vi "Trace Results.vi"(9 "Status of previous command":T1, 10 "Description":string, 11 "Subsystem":string) -> ()   [LabVIEW 2015]
doc: "This VI displays the execution trace of various commands and subsystems. Use command descriptions and controller print formatting to make it easier to understand the trace."
uses:
  <vilib>/Rock Robotics/WPI/Framework/Completion Status.ctl
panel:
  in  "Trace Enable":bool
  out "Subsystem Trace":T2(array[cluster])
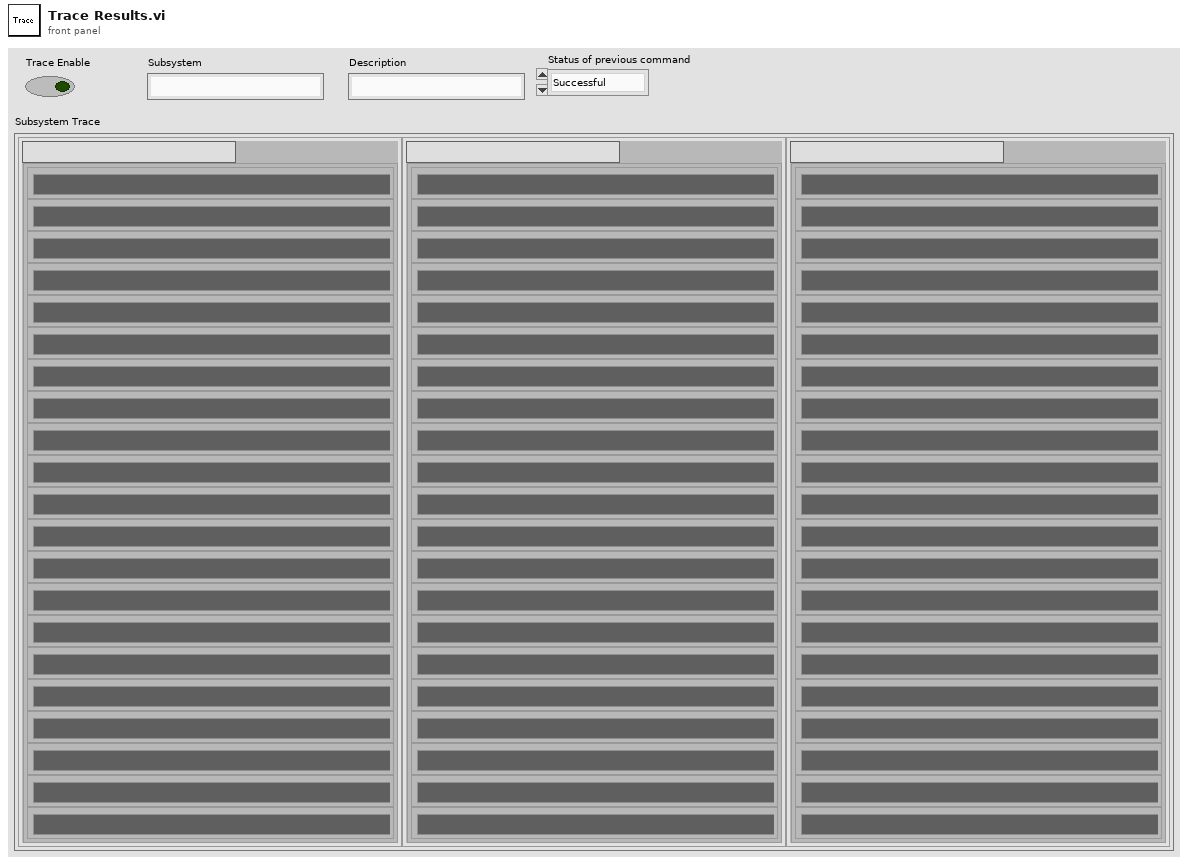
[diagram p1: front panel]
types:
  T1 = typedef "Completion Status.ctl" = enum16{"Successful", "Aborted", "Incomplete"}
  T2 = cluster{"Subsystem":string, "Tracings":cluster{"Command":string, "Color":u32}[]}[]
  T3 = cluster{"Subsystem":string, "Tracings":cluster{"Command":string, "Color":u32}[]}
  T4 = cluster{"Subsystem":string, cluster{"Description":string, "Active":u32}[]}
  T5 = cluster{"Subsystem":string, "Tracings":cluster{"Description":string, "Active":u32}[]}[]
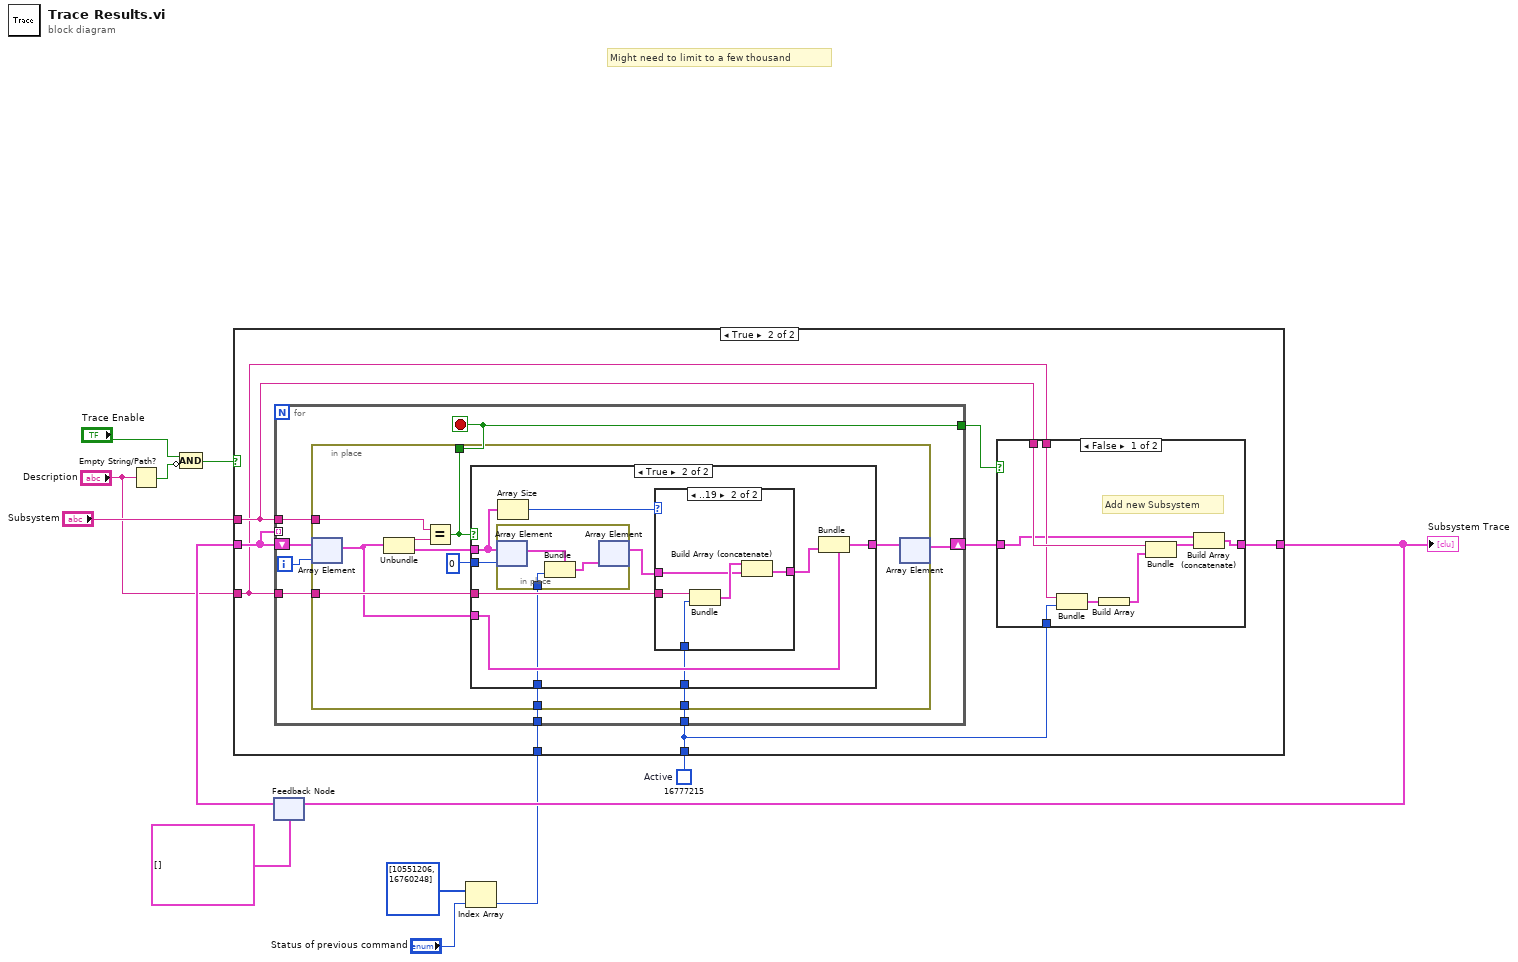
[diagram p0: block diagram]
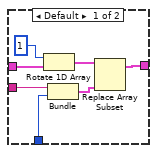
[diagram p5: hidden frame]
diagram:
  w7 = u32 16777215  # Active
  # "Might need to limit to a few thousand"
  n1 = Empty String/Path?(string/path="Description") -> (empty?=w12:bool)
  n2 = Compound Arithmetic op=AND("Trace Enable", invert w12) -> (w3:bool)
  n3 = feedback #1(T2 []) -> (w10:T2)
  n4 = Index Array(array=u32[] [10551206, 16760248], index="Status of previous command") -> (element=w2:u32)
  n5 = case shown="True" w3 {
    tunnel: w10 -> [w13 w21]
    tunnel: "Subsystem" -> [_ w18]
    tunnel: "Description" -> [_ w17]
    tunnel: w7 -> [_ w16]
    tunnel: [w13 w15] -> w6
    tunnel: w2 -> [_ w14]
    frame False {
    }
    frame True {
      n6 = for {
        tunnel: w18 -> [w38]
        tunnel: w17 -> [w37]
        shift-right: [w34] -> w19
        shift-left: w21 -> [w36]
        tunnel: [w33] -> w20
        tunnel: w21 -> [_] mode=indexing
        tunnel: w16 -> [w32]
        tunnel: w14 -> [w31]
        i -> [w35]
        stop <- w33 stop-if-true
        n7 = in-place {
          in-place-border: w38 -> [w47]
          in-place-border: w37 -> [w45]
          in-place-border: [w42] -> w33
          in-place-border: w32 -> [w41]
          in-place-border: w31 -> [w40]
          n8 = in-place-array #2(w36, w35) -> (w43:T3)
          n9 = Unbundle(w43) -> ("Subsystem"=w48:string, "Tracings"=w46:cluster{"Command":string, "Color":u32}[])
          n10 = Equal?(x=w47, y=w48) -> (x = y?=w42:bool)
          n11 = case shown="True" w42 {
            tunnel: w46 -> [_ w53]
            tunnel: w45 -> [_ w58]
            tunnel: [w49 w57] -> w44
            tunnel: w43 -> [w49 w56]
            tunnel: w41 -> [_ w54]
            tunnel: w40 -> [_ w51]
            tunnel: 0 -> [_ w50]
            frame False {
            }
            frame True {
              n12 = in-place {
                in-place-border: w51 -> [w60]
                n13 = in-place-array #3(w53, w50) -> (w62:cluster{"Command":string, "Color":u32})
                n14 = Bundle(cluster=w62, "Color"=w60) -> (w61:cluster{"Command":string, "Color":u32})  [unwired: 1 in]
                n15 = in-place-array #3(w61) -> (w52:cluster{"Command":string, "Color":u32}[])  [unwired: 1 out]
              }
              n16 = Array Size(array=w53) -> (size(s)=w59:i32)
              n17 = case shown="..19" w59 {
                tunnel: w52 -> [w69 w70]
                tunnel: w58 -> [w66 w73]
                tunnel: [w65 w74] -> w55
                tunnel: w54 -> [w63 w71]
                frame Default {
                  n18 = Rotate 1D Array(1:w69, 2:1 ("n")) -> (0:w67:cluster{"Command":string, "Color":u32}[])
                  n19 = Bundle("Description"=w66, "Active"=w63) -> (w64:cluster{"Description":string, "Active":u32})  [unwired: 1 in]
                  n20 = Replace Array Subset(array=w67, new element=w64) -> (w65:cluster{"Command":string, "Color":u32}[])  [unwired: 1 in]
                }
                frame ..19 {
                  n21 = Bundle("Description"=w73, "Active"=w71) -> (w72:cluster{"Description":string, "Active":u32})  [unwired: 1 in]
                  n22 = Build Array (concatenate)(w72, w70) -> (w74:cluster{"Command":string, "Color":u32}[])
                }
              }
              n23 = Bundle(cluster=w56, "Tracings"=w55) -> (w57:T3)  [unwired: 1 in]
            }
          }
          n24 = in-place-array #2(w44) -> (w34:T2)  [unwired: 1 out]
        }
      }
      n25 = case shown="False" w20 {
        tunnel: w19 -> [w22 w30]
        tunnel: [w24 w30] -> w15
        tunnel: w18 -> [w28 _]
        tunnel: w17 -> [w26 _]
        tunnel: w16 -> [w23 _]
        frame False {
          # "Add new Subsystem"
          n26 = Bundle("Description"=w26, "Active"=w23) -> (w29:cluster{"Description":string, "Active":u32})  [unwired: 1 in]
          n27 = Build Array(w29) -> (w27:cluster{"Description":string, "Active":u32}[])
          n28 = Bundle("Subsystem"=w28, w27) -> (w25:T4)  [unwired: 1 in]
          n29 = Build Array (concatenate)(w22, w25) -> (w24:T5)
        }
        frame True {
        }
      }
    }
  }
  "Subsystem Trace" <- w6
  n30 = feedback-in #1(w6) -> ()
